vi "read from web.vi"() -> ()   [LabVIEW 2018]
panel:
  out "before substring":string
  out "after substring":string
  out "error out 2":errorcluster
  in  "regular expression 2":string
  out "Array":string[](array[string])
  in  "regular expression In Loop":string
  in  "regular expression":string
  out "timed out":bool
  out "error out":errorcluster
  in  "error in (no error)":errorcluster
  in  "ms timeout (10000)":i32
  in  "mode":T1(ring)
  in  "URL":string
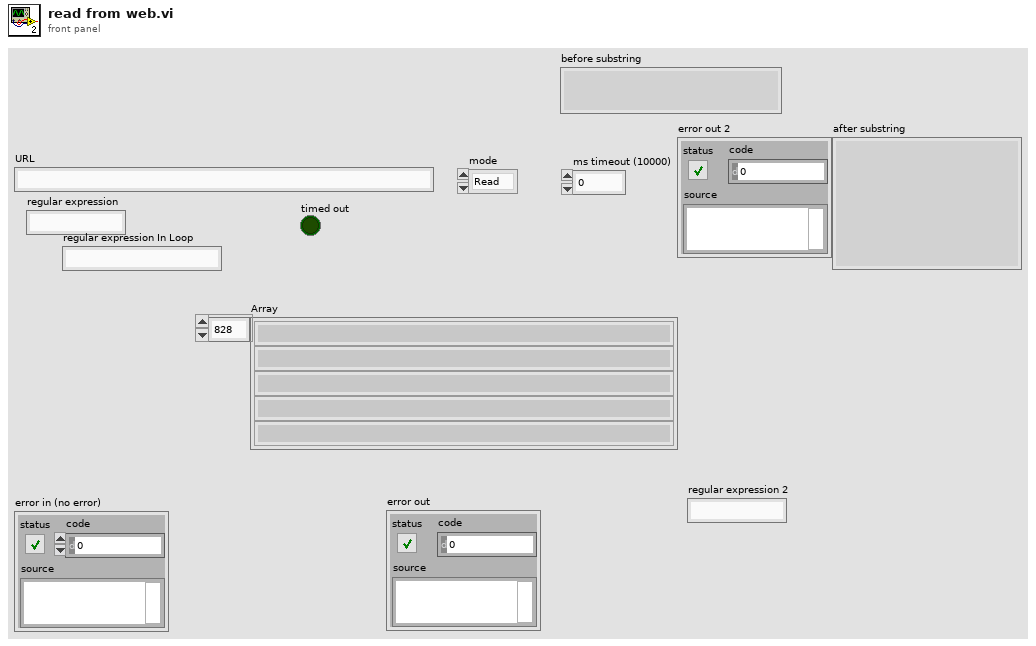
[diagram p1: front panel]
types:
  T1 = enum16{"Read", "Write", "ReadWrite", "BufferedRead", "BufferedReadWrite"}
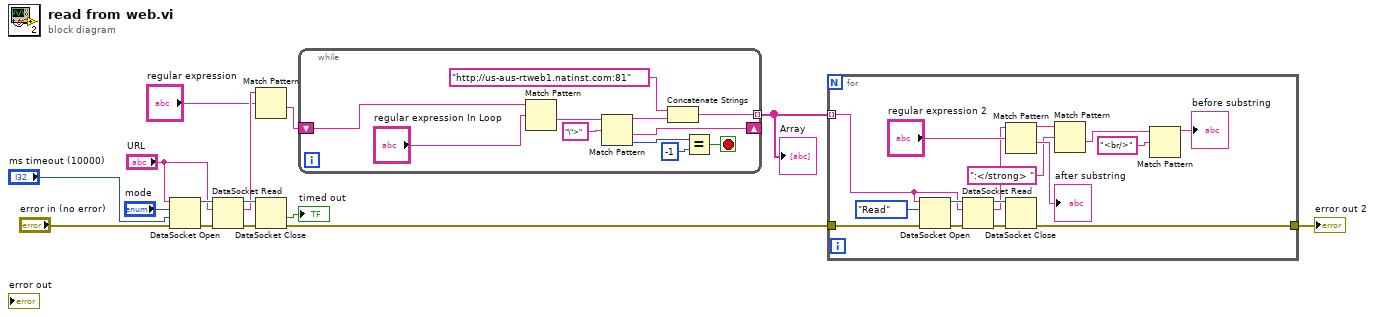
[diagram p0: block diagram]
diagram:
  n1 = DataSocket Open(8:"error in (no error)", 9:"ms timeout (10000)", 10:"mode", 11:"URL") -> (0:w15:errorcluster, 3:w9:refnum<k13>)
  n2 = DataSocket Read(8:w15, 10:"URL", 11:w9) -> (0:w14:errorcluster, 2:w6:string, 3:w7:refnum<k13>)  [unwired: 2 in, 4 out]
  n3 = Match Pattern(string=w6, regular expression="regular expression") -> (after substring=w4:string)  [unwired: 1 in, 3 out]
  n4 = DataSocket Close(8:w14, 11:w7) -> (0:w3:errorcluster, 1:→"timed out":bool)  [unwired: 1 in]
  n5 = while {
    tunnel: [w17] -> w2 mode=indexing
    shift-right: [w22] -> _
    shift-left: w4 -> [w26]
    stop <- w19 stop-if-true
    n6 = Match Pattern(string=w26, regular expression="regular expression In Loop") -> (after substring=w24:string)  [unwired: 1 in, 3 out]
    n7 = Match Pattern(string=w24, regular expression="\">") -> (before substring=w18:string, after substring=w22:string, offset past match=w21:i32)  [unwired: 1 in, 1 out]
    n8 = Concatenate Strings("http://us-aus-rtweb1.natinst.com:81" ("string"), w18) -> (w17:string)
    n9 = Equal?(x=w21, y=-1) -> (x = y?=w19:bool)
  }
  "Array" <- w2
  n10 = for {
    tunnel: w3 -> [w37]
    tunnel: w2 -> [w36] mode=indexing
    tunnel: [w35] -> w1
    n11 = DataSocket Open(8:w37, 10:T1."Read" ("mode"), 11:w36) -> (0:w42:errorcluster, 3:w40:refnum<k13>)  [unwired: 1 in]
    n12 = DataSocket Read(8:w42, 10:w36, 11:w40) -> (0:w41:errorcluster, 2:w32:string, 3:w39:refnum<k13>)  [unwired: 2 in, 4 out]
    n13 = Match Pattern(string=w32, regular expression="regular expression 2") -> (before substring=w30:string, after substring=→"after substring":string)  [unwired: 1 in, 2 out]
    n14 = DataSocket Close(8:w41, 11:w39) -> (0:w35:errorcluster)  [unwired: 1 in, 1 out]
    n15 = Match Pattern(string=w30, regular expression=":</strong> ") -> (after substring=w29:string)  [unwired: 1 in, 3 out]
    n16 = Match Pattern(string=w29, regular expression="<br/>") -> (before substring=→"before substring":string)  [unwired: 1 in, 3 out]
  }
  "error out 2" <- w1
